vi "GetAdapters.vi"(8 "error in":errorcluster) -> (0 "error out":errorcluster, 3 "AdaptersOut":T1[](array[typedef]))   [LabVIEW 2011, in "Konvolucio MUDS150628.lvlib"]
uses:
  <instrlib>/Konvolucio MCAN120803/Types/AdapterItemType.ctl
  C:/Program Files/National Instruments/LabVIEW 2011/instr.lib/Konvolucio MCAN120803/Private/Konvolucio.MCAN120803.dll
  Konvolucio MCAN120803/Private/Konvolucio.MCAN120803.dll
  <instrlib>/Konvolucio MUDS150628/Konvolucio MUDS150628.lvlib
  <instrlib>/Konvolucio MCAN120803/Konvolucio MCAN120803.lvlib
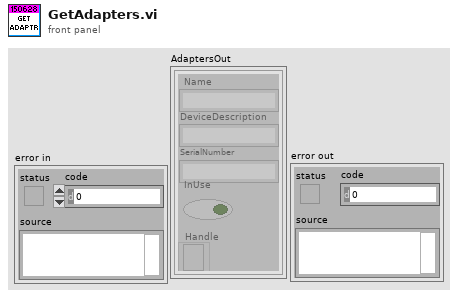
[diagram p1: front panel]
types:
  T1 = typedef "Konvolucio MCAN120803.lvlib/AdapterItemType.ctl" = cluster{"Name":string, "DeviceDescription":string, "SerialNumber":string, "InUse":bool, "Handle":refnum<k24>}
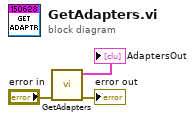
[diagram p0: block diagram]
diagram:
  n1 = call <instrlib>:"GetAdapters.vi"("error in"="error in") -> ("error out"=→"error out":errorcluster, "AdaptersOut"=→"AdaptersOut":T1[])  [unwired: 9 in]
